vi "Run Framework Configuration.vi"() -> ()   [LabVIEW 2019]
uses:
  <vilib>/NI/Memory Manager/Classes/Pointer/Pointer.lvclass
  <vilib>/NI/Memory Manager/Classes/Pointer/Write U32.vi
  <vilib>/NI/Memory Manager/Classes/Pointer/Write Bool.vi
  <vilib>/NI/Memory Manager/Classes/Pointer/Read Bool.vi
  <vilib>/NI/Memory Manager/Classes/Pointer/Read I32.vi
  <vilib>/NI/Memory Manager/Classes/Pointer/Read U32.vi
  SubVIs/UI Pointers.ctl
  <vilib>/addons/VeriStand Custom Device Scripting APIs/Data Sharing Framework/DSF Core.lvlibp/Typedefs/DSF Timing Info.ctl
  <vilib>/addons/VeriStand Custom Device Scripting APIs/Data Sharing Framework/DSF Core.lvlibp
  <vilib>/addons/VeriStand Custom Device Scripting APIs/Data Sharing Framework/DSF Core.lvlibp/Typedefs/DSF Direction.ctl
  <vilib>/addons/VeriStand Custom Device Scripting APIs/Data Sharing Framework/DSF Core.lvlibp/Typedefs/DSF Data Type.ctl
  <vilib>/addons/VeriStand Custom Device Scripting APIs/Data Sharing Framework/DSF Core.lvlibp/Typedefs/DSF Engine Channel Configuration.ctl
  <vilib>/addons/VeriStand Custom Device Scripting APIs/Data Sharing Framework/DSF Core.lvlibp/Typedefs/DSF Settings Info.ctl
  <vilib>/addons/VeriStand Custom Device Scripting APIs/Data Sharing Framework/DSF Core.lvlibp/Typedefs/DSF Engine Transfer Configuration.ctl
  <vilib>/addons/VeriStand Custom Device Scripting APIs/Data Sharing Framework/DSF Core.lvlibp/Typedefs/DSF Engine Transfer Group Configuration.ctl
  <vilib>/addons/VeriStand Custom Device Scripting APIs/Data Sharing Framework/DSF Core.lvlibp/Typedefs/DSF Engine Plugin Configuration.ctl
  <vilib>/addons/VeriStand Custom Device Scripting APIs/Data Sharing Framework/DSF Core.lvlibp/Typedefs/DSF Engine Framework Configuration.ctl
  <vilib>/addons/VeriStand Custom Device Scripting APIs/Data Sharing Framework/DSF Core.lvlibp/Classes/Framework/Framework Options.ctl
  <vilib>/addons/VeriStand Custom Device Scripting APIs/Data Sharing Framework/DSF Core.lvlibp/Classes/Framework/Framework.lvclass
  <vilib>/addons/VeriStand Custom Device Scripting APIs/Data Sharing Framework/DSF Core.lvlibp/Typedefs/DSF Engine Plugin Thread Configuration.ctl
  <vilib>/addons/VeriStand Custom Device Scripting APIs/Data Sharing Framework/DSF Core.lvlibp/Typedefs/DSF Timeout Behavior.ctl
  <vilib>/addons/VeriStand Custom Device Scripting APIs/Data Sharing Framework/DSF Core.lvlibp/Typedefs/DSF Performance Options.ctl
  <vilib>/addons/VeriStand Custom Device Scripting APIs/Data Sharing Framework/DSF Core.lvlibp/Typedefs/DSF FIFO Options.ctl
  <vilib>/addons/VeriStand Custom Device Scripting APIs/Data Sharing Framework/DSF Core.lvlibp/Classes/Thread/Thread Options.ctl
  <vilib>/addons/VeriStand Custom Device Scripting APIs/Data Sharing Framework/DSF Core.lvlibp/Classes/Thread/Thread.lvclass
  <vilib>/addons/VeriStand Custom Device Scripting APIs/Data Sharing Framework/DSF Core.lvlibp/Typedefs/DSF Plugin Options.ctl
  <vilib>/addons/VeriStand Custom Device Scripting APIs/Data Sharing Framework/DSF Core.lvlibp/Classes/Framework/Data Server Options.ctl
  <vilib>/addons/VeriStand Custom Device Scripting APIs/Data Sharing Framework/DSF Core.lvlibp/Typedefs/Core Plugin Configuration.ctl
  <vilib>/addons/VeriStand Custom Device Scripting APIs/Data Sharing Framework/DSF Core.lvlibp/Classes/Configuration/Core/Plugin/Plugin Configuration.lvclass
  <vilib>/addons/VeriStand Custom Device Scripting APIs/Data Sharing Framework/DSF Core.lvlibp/Typedefs/Core Thread Configuration.ctl
  <vilib>/addons/VeriStand Custom Device Scripting APIs/Data Sharing Framework/DSF Core.lvlibp/Classes/Configuration/Core/Thread/Thread Configuration.lvclass
  <vilib>/addons/VeriStand Custom Device Scripting APIs/Data Sharing Framework/DSF Core.lvlibp/Typedefs/Core Group Configuration.ctl
  <vilib>/addons/VeriStand Custom Device Scripting APIs/Data Sharing Framework/DSF Core.lvlibp/Classes/Configuration/Core/Group/Group Configuration.lvclass
  <vilib>/addons/VeriStand Custom Device Scripting APIs/Data Sharing Framework/DSF Core.lvlibp/Typedefs/Core Transfer Configuration.ctl
  <vilib>/addons/VeriStand Custom Device Scripting APIs/Data Sharing Framework/DSF Core.lvlibp/Classes/Configuration/Core/Transfer/Transfer Configuration.lvclass
  <vilib>/addons/VeriStand Custom Device Scripting APIs/Data Sharing Framework/DSF Core.lvlibp/Typedefs/Core Channel Configuration.ctl
  <vilib>/addons/VeriStand Custom Device Scripting APIs/Data Sharing Framework/DSF Core.lvlibp/Classes/Configuration/Core/Channel/Channel Configuration.lvclass
panel:
  in  "thread settings":cluster{"Processor":i32, "Priority":i32}={"Processor"=-2, "Priority"=100}
  out "framework configuration":T1
  out "actual frequency":u32 format="%.0pHz"
  in  "target frequency":u32=100 format="%.0pHz"
  in  "components directory":path
  in  "dsf configuration file path":path=path "C:/Users/Admin/Desktop/test.dsf"
  out "iteration":i32
  out "error out":errorcluster
  in  "framework options":T17={"FIFO Options"={"Infinite Timeouts"=FALSE}, "Thread Options"={"Show FP On Call"=TRUE, "Close FP After Call"=TRUE, "Allow Debugging"=TRUE}, "Plugin Options"={"Default Components"=TRUE}, "Performance Options"={"Measure Period"=TRUE, "Measure Rx/Tx Duration"=TRUE}, "Data Server Options"={"Enable Data Server"=FALSE, "Period"=50}} {"Data Server Options"."Period" format="%d ms"}
  in  "stop":bool
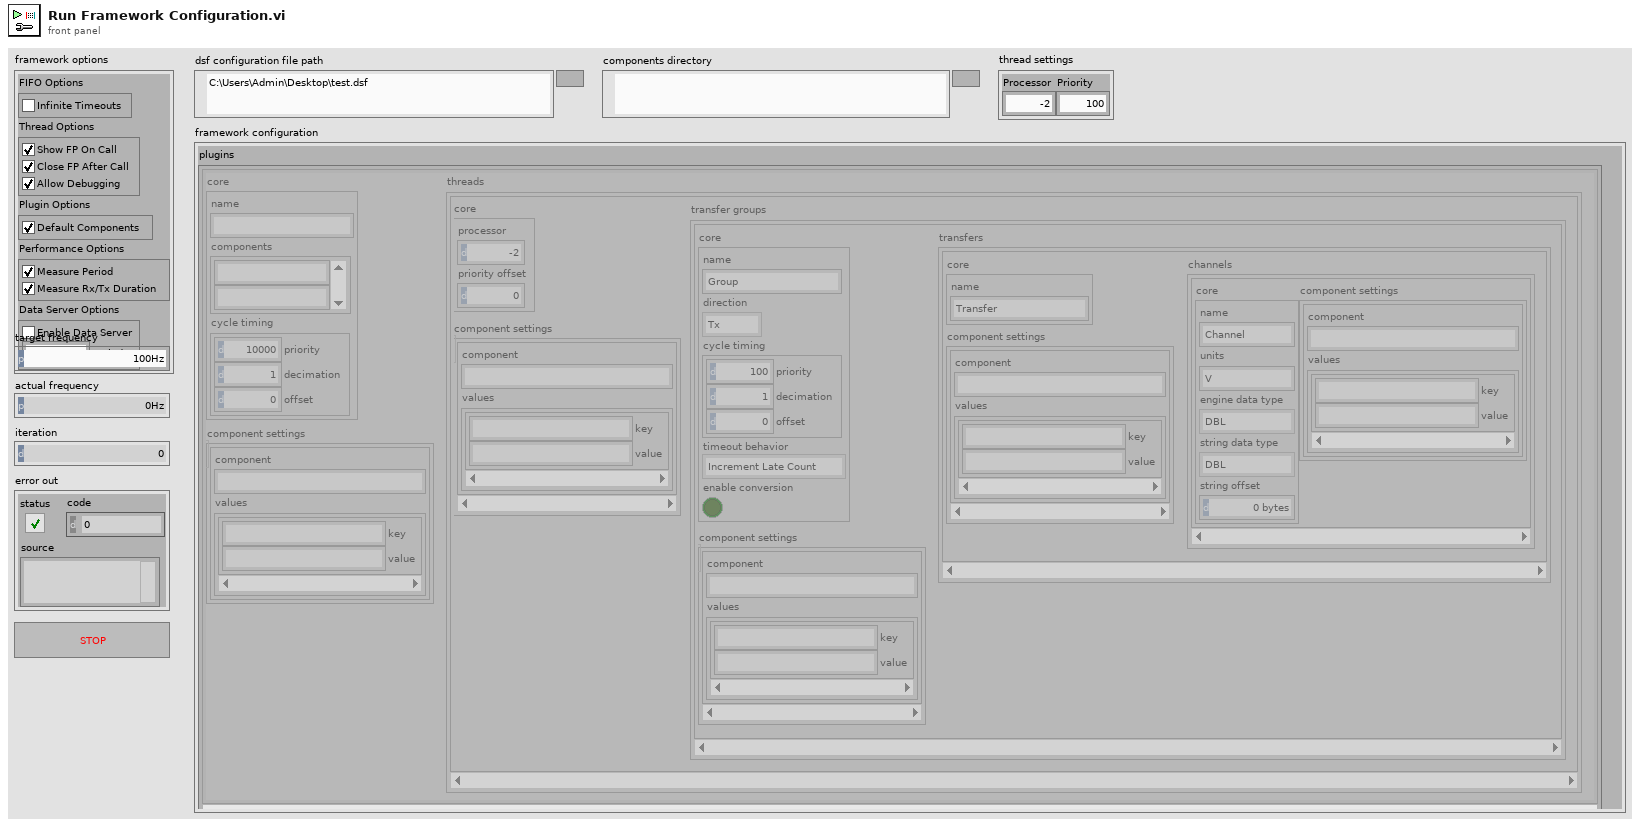
[diagram p1: front panel]
types:
  T1 = typedef "DSF Core.lvlibp/DSF Engine Framework Configuration.ctl" = cluster{"plugins":T2[]}
  T2 = typedef "DSF Core.lvlibp/DSF Engine Plugin Configuration.ctl" = cluster{"core":T3, "component settings":T5[], "threads":T6[]}
  T3 = typedef "DSF Core.lvlibp/Plugin Configuration.lvclass/Core Plugin Configuration.ctl" = cluster{"name":string, "components":string[], "cycle timing":T4}
  T4 = typedef "DSF Core.lvlibp/DSF Timing Info.ctl" = cluster{"priority":u64, "decimation":u64, "offset":u64}
  T5 = typedef "DSF Core.lvlibp/DSF Settings Info.ctl" = cluster{"component":string, "values":cluster{"key":string, "value":string}[]}
  T6 = typedef "DSF Core.lvlibp/DSF Engine Plugin Thread Configuration.ctl" = cluster{"core":T7, "component settings":T5[], "transfer groups":T8[]}
  T7 = typedef "DSF Core.lvlibp/Thread Configuration.lvclass/Core Thread Configuration.ctl" = cluster{"processor":i32, "priority offset":i16}
  T8 = typedef "DSF Core.lvlibp/DSF Engine Transfer Group Configuration.ctl" = cluster{"core":T9, "component settings":T5[], "transfers":T12[]}
  T9 = typedef "DSF Core.lvlibp/Group Configuration.lvclass/Core Group Configuration.ctl" = cluster{"name":string, "direction":T10, "cycle timing":T4, "timeout behavior":T11, "enable conversion":bool}
  T10 = typedef "DSF Core.lvlibp/DSF Direction.ctl" = enum8{"Tx", "Rx"}
  T11 = typedef "DSF Core.lvlibp/DSF Timeout Behavior.ctl" = enum8{"Increment Late Count", "Throw Error"}
  T12 = typedef "DSF Core.lvlibp/DSF Engine Transfer Configuration.ctl" = cluster{"core":T13, "component settings":T5[], "channels":T14[]}
  T13 = typedef "DSF Core.lvlibp/Transfer Configuration.lvclass/Core Transfer Configuration.ctl" = cluster{"name":string}
  T14 = typedef "DSF Core.lvlibp/DSF Engine Channel Configuration.ctl" = cluster{"core":T15, "component settings":T5[]}
  T15 = typedef "DSF Core.lvlibp/Channel Configuration.lvclass/Core Channel Configuration.ctl" = cluster{"name":string, "units":string, "engine data type":T16, "string data type":T16, "string offset":u64}
  T16 = typedef "DSF Core.lvlibp/DSF Data Type.ctl" = enum8{"Bool", "SGL", "DBL", "I8", "I16", "I32", "I64", "U8", "U16", "U32", "U64"}
  T17 = typedef "DSF Core.lvlibp/Framework.lvclass/Framework Options.ctl" = cluster{"FIFO Options":T18, "Thread Options":T19, "Plugin Options":T20, "Performance Options":T21, "Data Server Options":T22}
  T18 = typedef "DSF Core.lvlibp/Framework.lvclass/DSF FIFO Options.ctl" = cluster{"Infinite Timeouts":bool}
  T19 = typedef "DSF Core.lvlibp/Thread.lvclass/Thread Options.ctl" = cluster{"Show FP On Call":bool, "Close FP After Call":bool, "Allow Debugging":bool}
  T20 = typedef "DSF Core.lvlibp/Framework.lvclass/DSF Plugin Options.ctl" = cluster{"Default Components":bool}
  T21 = typedef "DSF Core.lvlibp/DSF Performance Options.ctl" = cluster{"Measure Period":bool, "Measure Rx/Tx Duration":bool}
  T22 = typedef "DSF Core.lvlibp/Framework.lvclass/Data Server Options.ctl" = cluster{"Enable Data Server":bool, "Period":u32}
  T23 = typedef "UI Pointers.ctl" = cluster{"Stop":refnum<class "Pointer.lvclass">, "Target Period":refnum<class "Pointer.lvclass">, "Actual Period":refnum<class "Pointer.lvclass">, "Iteration":refnum<class "Pointer.lvclass">}
  T24 = typedef "DSF Core.lvlibp/DSF Engine Framework Configuration.ctl" = cluster{"Plugins":T25[]}
  T25 = typedef "DSF Core.lvlibp/DSF Engine Plugin Configuration.ctl" = cluster{"name":string, "components":string[], "cycle timing":T4, "threads":T26[], "Transfer Groups":T28[], "settings":T27}
  T26 = typedef "DSF Core.lvlibp/DSF Engine Plugin Thread Configuration.ctl" = cluster{"buffer converter settings":T27, "transceiver settings":T27, "custom settings":T27, "processor":i32, "priority offset":i16}
  T27 = typedef "DSF Core.lvlibp/DSF Settings Info.ctl" = cluster{"key":string, "value":string}[]
  T28 = typedef "DSF Core.lvlibp/DSF Engine Transfer Group Configuration.ctl" = cluster{"name":string, "direction":T10, "cycle timing":T4, "thread index":i32, "settings":T27, "Transfers":T29[], "timeout behavior":T11}
  T29 = typedef "DSF Core.lvlibp/DSF Engine Transfer Configuration.ctl" = cluster{"name":string, "byte order":T30, "settings":T27, "channels":T31[]}
  T30 = typedef "DSF Core.lvlibp/DSF Byte Order.ctl" = enum8{"big-endian", "little-endian"}
  T31 = typedef "DSF Core.lvlibp/DSF Engine Channel Configuration.ctl" = cluster{"string offset":u64, "string data type":T16, "engine data type":T16, "name":string, "settings":T27, "units":string}
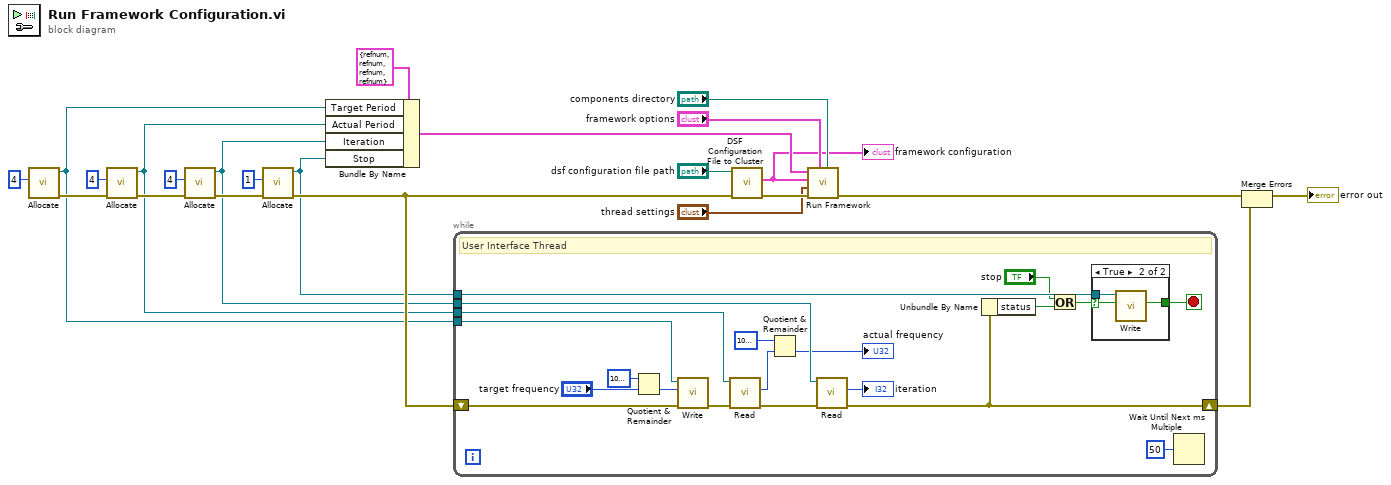
[diagram p0: block diagram]
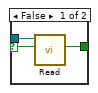
[diagram p2: hidden frame]
diagram:
  n1 = call <vilib>:"Allocate.vi"("size"=u64 4) -> ("error out"=w16:errorcluster, "Pointer out"=w8:refnum<class "Pointer.lvclass">)  [unwired: 9 in]
  n2 = call <vilib>:"Allocate.vi"("error in (no error)"=w16, "size"=u64 4) -> ("error out"=w18:errorcluster, "Pointer out"=w9:refnum<class "Pointer.lvclass">)  [unwired: 8 in]
  n3 = call <vilib>:"Allocate.vi"("error in (no error)"=w18, "size"=u64 4) -> ("error out"=w13:errorcluster, "Pointer out"=w10:refnum<class "Pointer.lvclass">)  [unwired: 8 in]
  n4 = call <vilib>:"Allocate.vi"("error in (no error)"=w13, "size"=u64 1) -> ("error out"=w23:errorcluster, "Pointer out"=w6:refnum<class "Pointer.lvclass">)  [unwired: 8 in]
  n5 = Bundle By Name(cluster=T23 {"Stop"=refnum, "Target Period"=refnum, "Actual Period"=refnum, "Iteration"=refnum} ("user interface pointers (null)"), "Target Period"=w8, "Actual Period"=w9, "Iteration"=w10, "Stop"=w6) -> (w2:T23)
  n6 = while {
    tunnel: w6 -> [w43]
    shift-right: [w32] -> w11
    shift-left: w23 -> [w39]
    tunnel: w8 -> [w36]
    tunnel: w9 -> [w34]
    tunnel: w10 -> [w31]
    stop <- w42 stop-if-true
    # "User Interface Thread"
    n7 = Quotient & Remainder(x=u32 1000000 ("y"), y="target frequency") -> (floor(x/y)=w35:u32)  [unwired: 1 out]
    n8 = call-poly <vilib>:"Write.vi"("error in (no error)"=w39, "value"=w35, "Pointer in"=w36) -> ("error out"=w37:errorcluster)  [unwired: 5 in, 3 out]
    n9 = call-poly <vilib>:"Read.vi"("error in (no error)"=w37, "Pointer in"=w34) -> ("error out"=w33:errorcluster, "value out"=w28:u32)  [unwired: 6 in, 2 out]
    n10 = Quotient & Remainder(x=u32 1000000 ("y"), y=w28) -> (floor(x/y)=→"actual frequency":u32)  [unwired: 1 out]
    n11 = call-poly <vilib>:"Read.vi"("error in (no error)"=w33, "Pointer in"=w31) -> ("error out"=w32:errorcluster, "value out"=→"iteration":i32)  [unwired: 6 in, 2 out]
    n12 = Unbundle By Name(w32) -> ("status"=w40:bool)
    n13 = Or(x="stop", y=w40) -> (x .or. y?=w41:bool)
    n14 = case shown="True" w41 {
      selector: w41 -> [w45 w48]
      tunnel: w43 -> [w46 w49]
      tunnel: [w44 w47] -> w42
      frame False {
        n15 = call-poly <vilib>:"Read.vi"("value in"=w45, "Pointer in"=w46) -> ("value out"=w44:bool)  [unwired: 6 in, 3 out]
      }
      frame True {
        n16 = call-poly <vilib>:"Write.vi"("value"=w48, "Pointer in"=w49) -> ("value"=w47:bool)  [unwired: 6 in, 3 out]
      }
    }
    n17 = Wait Until Next ms Multiple(millisecond multiple=u32 50) -> ()  [unwired: 1 out]
  }
  n18 = call "DSF Configuration File to Cluster.vi"("error in (no error)"=w23, "dsf configuration file path"="dsf configuration file path") -> ("error out"=w7:errorcluster, "framework configuration out"=w1:T24)  [unwired: 7 in, 1 out]
  "framework configuration" <- w1
  n19 = call "Run Framework.vi"("components directory"="components directory", "framework options"="framework options", "error in (no error)"=w7, "thread settings"="thread settings", "framework configuration"=w1, "user interface pointers (null)"=w2) -> ("error out"=w15:errorcluster)  [unwired: 5 in]
  n20 = Merge Errors(w15, w11) -> (→"error out":errorcluster)
